vi "Write Chirp.vi"(8 "error in (no error)":errorcluster, 10 "Chirp":cluster{"f_center":dbl, "bandwidth":dbl}={"f_center"=1350.0, "bandwidth"=150.0}, 11 "PAS in":refnum<class "PAS.lvclass">) -> (0 "error out":errorcluster, 3 "PAS out":refnum<class "PAS.lvclass">)   [LabVIEW 2016, in "PAS Library.lvlib" / "PAS.lvclass"]
uses:
  PAS.lvclass
  PAS.lvclass/PAS.ctl
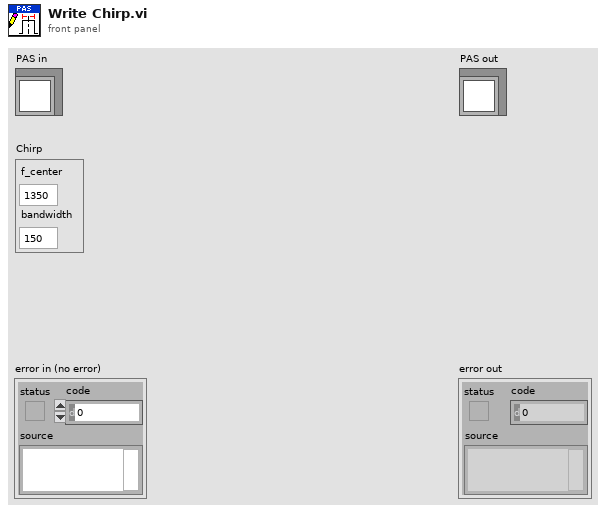
[diagram p1: front panel]
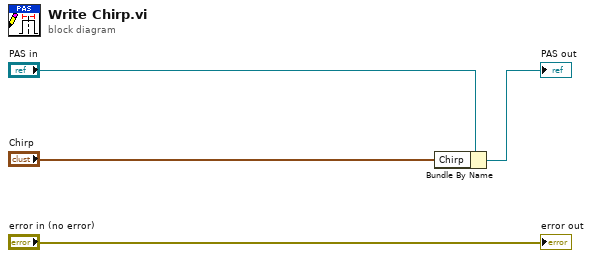
[diagram p0: block diagram]
diagram:
  n1 = Bundle By Name(cluster="PAS in", "Chirp"="Chirp") -> (→"PAS out":refnum<class "PAS.lvclass">)
  "error out" <- "error in (no error)"
